vi "Read State.vi"(11 "Pump_1AI_1DO_2DI in":refnum<class "NeedleValve.lvclass">) -> (2 "StateValveModbus":T1=enum."OPEN")   [LabVIEW 2019, in "NeedleValve.lvclass"]
uses:
  NeedleValve.lvclass
  TypeDef/StateValveModbus.ctl
  NeedleValve.lvclass/NeedleValve.ctl
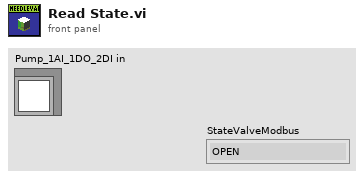
[diagram p1: front panel]
types:
  T1 = typedef "StateValveModbus.ctl" = enum16{"IDLE", "OPEN", "CLOSE", "OPENING", "CLOSING", "STOP"}
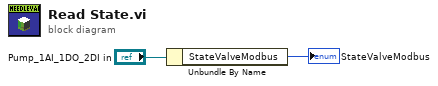
[diagram p0: block diagram]
diagram:
  n1 = Unbundle By Name("Pump_1AI_1DO_2DI in") -> ("StateValveModbus"=→"StateValveModbus":T1)
